vi "Write TDMS.vi"(8 "error in (no error)":errorcluster, 10 "path":path, 11 "LVtoITX in":refnum<class "LVtoITX.lvclass">) -> (0 "error out":errorcluster, 3 "LVtoITX out":refnum<class "LVtoITX.lvclass">)   [LabVIEW 2016, in "LVtoITX.lvclass"]
uses:
  LVtoITX.lvclass
  LVtoITX.lvclass/LVtoITX.ctl
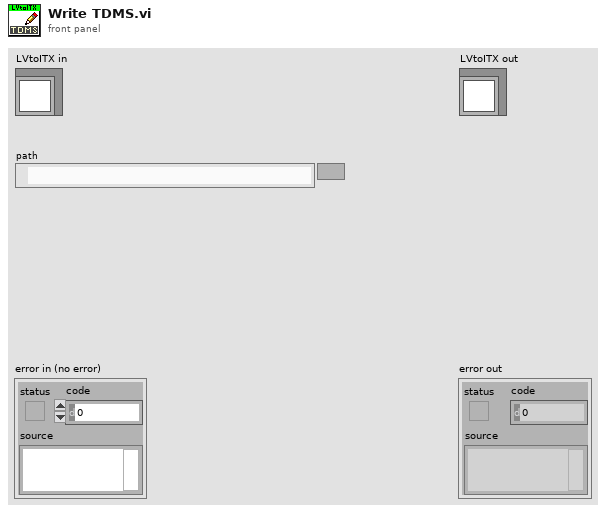
[diagram p1: front panel]
types:
  T1 = enum16{"open", "open or create", "create or replace", "create", "open (read-only)"}
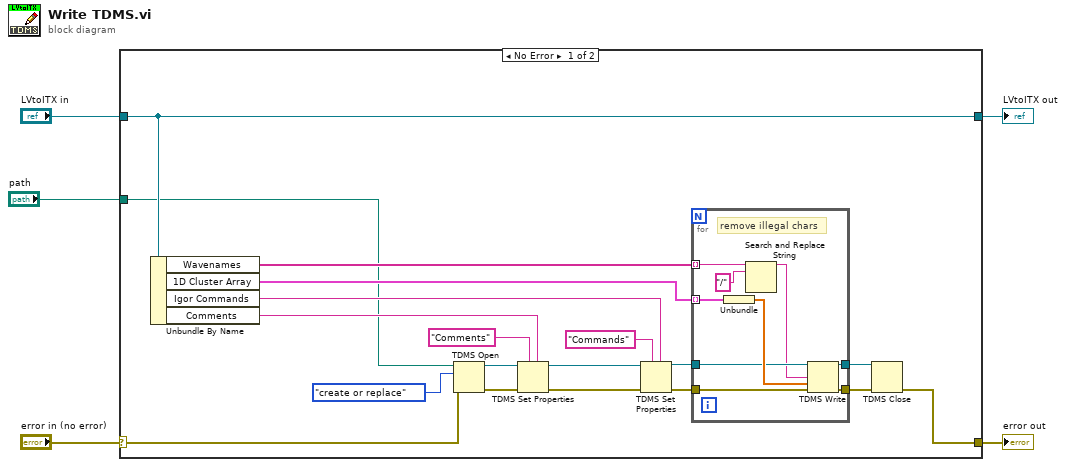
[diagram p0: block diagram]
diagram:
  n1 = case shown="No Error" "error in (no error)" {
    selector: "error in (no error)" -> [w10 w34]
    tunnel: [w14 w34] -> w2
    tunnel: [w24 w35] -> w3
    tunnel: "LVtoITX in" -> [w24 w35]
    tunnel: "path" -> [w6 _]
    frame No Error {
      n2 = Unbundle By Name(w24) -> ("Wavenames"=w9:string[], "1D Cluster Array"=w8:cluster{"array type (2D Dbl)":dbl[]}[], "Igor Commands"=w11:string, "Comments"=w12:string)
      n3 = TDMS Open(8:w10, 10:T1."create or replace" ("operation (0:open)"), 11:w6) -> (0:w23:errorcluster, 3:w22:refnum<k34>)  [unwired: 4 in]
      n4 = TDMS Set Properties(5:w12, 7:"Comments" ("attrib name"), 8:w23, 11:w22) -> (0:w18:errorcluster, 3:w19:refnum<k34>)  [unwired: 2 in, 2 out]
      n5 = TDMS Set Properties(5:w11, 7:"Commands" ("attrib name"), 8:w18, 11:w19) -> (0:w17:errorcluster, 3:w16:refnum<k34>)  [unwired: 2 in, 2 out]
      n6 = for {
        tunnel: w9 -> [w32] mode=indexing
        tunnel: w8 -> [w33] mode=indexing
        tunnel: w17 -> [w30]
        tunnel: w16 -> [w28]
        tunnel: [w27] -> w15
        tunnel: [w26] -> w13
        # "remove illegal chars"
        n7 = Unbundle(w33) -> ("array type (2D Dbl)"=w29:dbl[])
        n8 = Search and Replace String(input string=w32, search string="/") -> (result string=w25:string)  [unwired: 6 in, 3 out]
        n9 = TDMS Write(0:w28, 7:w25, 9:w29, 11:w30) -> (4:w26:refnum<k34>, 15:w27:errorcluster)  [unwired: 2 in, 2 out]
      }
      n10 = TDMS Close(8:w15, 11:w13) -> (0:w14:errorcluster)  [unwired: 1 out]
    }
    frame Error {
    }
  }
  "error out" <- w2
  "LVtoITX out" <- w3
